vi "close connection.vi"() -> ()   [LabVIEW 2011]
panel:
  in  "VISA resource name":refnum<visa-resource-name>="COM8"
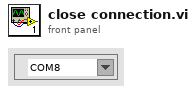
[diagram p1: front panel]
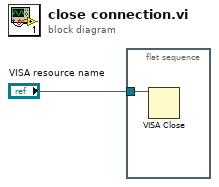
[diagram p0: block diagram]
diagram:
  n1 = flat-sequence {
    tunnel: "VISA resource name" -> [w2]
    frame #0 {
      n2 = VISA Close(VISA resource name=w2) -> ()  [unwired: 1 in, 1 out]
    }
  }
